vi "svc_Check Frequency Range.vi"(6 "effective band":cluster{"fl":dbl, "fh":dbl}={"fl"=0.0, "fh"=0.5} {"fh" format="%.2f"; "fl" format="%.2f"}, 7 "fs":dbl format="%.2f", 8 "error in (no error)":errorcluster, 9 "fmax":dbl=inf, 10 "f0":dbl, 11 "frequency range in":T1={"start frequency"=20.0, "stop frequency"=20000.0} {"stop frequency" format="%.2f"; "start frequency" format="%.2f"}) -> (0 "error out":errorcluster, 1 "frequency range changed":bool, 3 "frequency range out":T1={"start frequency"=20.0, "stop frequency"=20000.0} {"stop frequency" format="%.2f"; "start frequency" format="%.2f"})   [LabVIEW 2017]
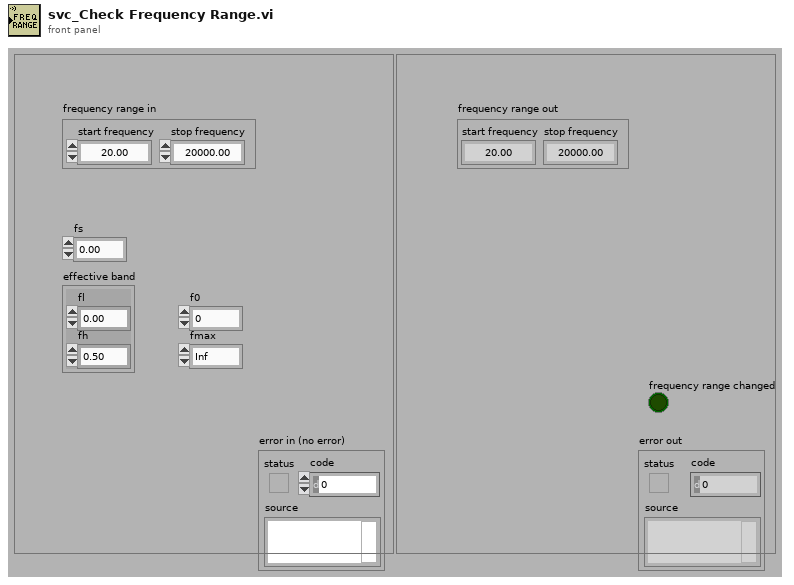
[diagram p1: front panel]
types:
  T1 = cluster{"start frequency":dbl, "stop frequency":dbl}
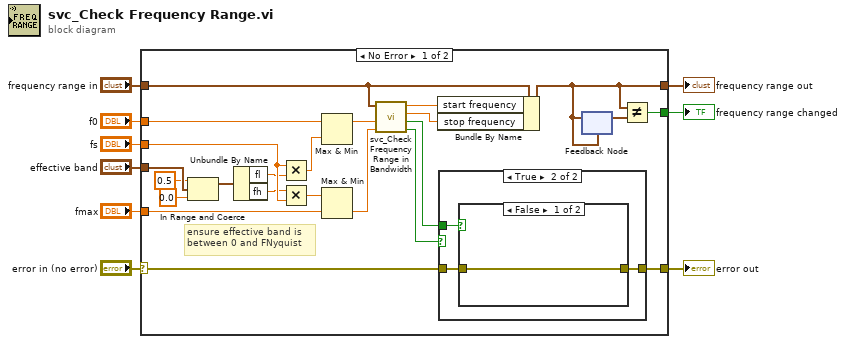
[diagram p0: block diagram]
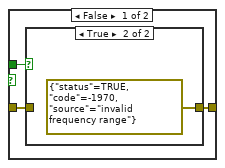
[diagram p2: hidden frame]
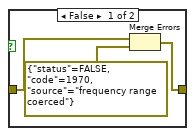
[diagram p3: hidden frame]
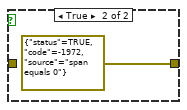
[diagram p4: hidden frame]
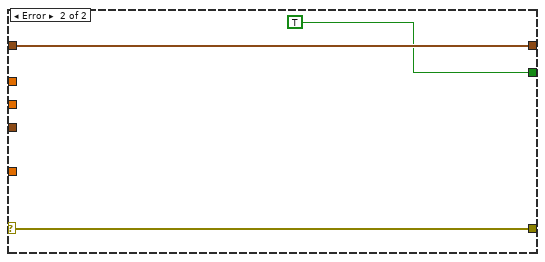
[diagram p5: hidden frame]
diagram:
  n1 = case shown="No Error" "error in (no error)" {
    selector: "error in (no error)" -> [w29 w47]
    tunnel: "effective band" -> [w32 _]
    tunnel: [w31 w47] -> w8
    tunnel: "fs" -> [w30 _]
    tunnel: "frequency range in" -> [w27 w46]
    tunnel: [w13 w46] -> w4
    tunnel: [w28 TRUE] -> w3
    tunnel: "f0" -> [w26 _]
    tunnel: "fmax" -> [w25 _]
    frame No Error {
      # "ensure effective band is\nbetween 0 and FNyquist"
      n2 = In Range and Coerce(upper limit=0.5 ("fs"), x=w32, lower limit=0.0 ("fs")) -> (coerced(x)=w12:cluster{"fl":dbl, "fh":dbl})  [unwired: 1 out]
      n3 = Unbundle By Name(w12) -> ("fl"=w24:dbl, "fh"=w23:dbl)
      n4 = Multiply(x=w30, y=w24) -> (x*y=w19:dbl)
      n5 = Multiply(x=w23, y=w30) -> (x*y=w17:dbl)
      n6 = Max & Min(x=w26, y=w19) -> (max(x,y)=w18:dbl)  [unwired: 1 out]
      n7 = Max & Min(x=w17, y=w25) -> (min(x,y)=w16:dbl)  [unwired: 1 out]
      n8 = call <vilib>:"svc_Check Frequency Range in Bandwidth.vi"("fmax"=w16, "fmin"=w18, "frequency range"=w27) -> ("start and stop in range"=w15:bool, "zero span"=w22:bool, "stop frequency"=w20:dbl, "start frequency"=w21:dbl)  [unwired: 5 in]
      n9 = Bundle By Name(cluster=w27, "start frequency"=w21, "stop frequency"=w20) -> (w13:T1)
      n10 = case shown="True" w15 {
        tunnel: [w34 w41] -> w31
        tunnel: w29 -> [w33 w40]
        tunnel: w22 -> [w35 w42]
        frame False {
          n11 = case shown="True" w35 {
            tunnel: [w36 errorcluster {"status"=TRUE, "code"=-1970, "source"="invalid frequency range"} ("error in (no error)")] -> w34
            tunnel: w33 -> [w38 _]
            frame False {
              n12 = Merge Errors(w38, errorcluster {"status"=FALSE, "code"=1970, "source"="frequency range coerced"} ("error in (no error)")) -> (w36:errorcluster)
            }
            frame True {
            }
          }
        }
        frame True {
          n13 = case shown="False" w42 {
            tunnel: [w43 errorcluster {"status"=TRUE, "code"=-1972, "source"="span equals 0"} ("error out")] -> w41
            tunnel: w40 -> [w43 _]
            frame False {
            }
            frame True {
            }
          }
        }
      }
      n14 = feedback #1(w13) -> (w14:T1)
      n15 = feedback-in #1(w13) -> ()
      n16 = Not Equal?(x=w13, y=w14) -> (x != y?=w28:bool)
    }
    frame Error {
    }
  }
  "error out" <- w8
  "frequency range out" <- w4
  "frequency range changed" <- w3
